vi "Error Query.vi"(8 "error in (no error)":errorcluster, 11 "VISA resource name":refnum<visa-resource-name>) -> (0 "error out":errorcluster, 1 "Error Message":string, 2 "Error Code":i32[](array[numeric]), 3 "VISA resource name out":refnum<visa-resource-name>)   [LabVIEW 2025]
doc: "Queries the instrument for any errors in the instrument's error queue. It will continue to read errors until all errors have been read from the instrument. Any errors will be returned in the <B>error out</B> control.\n\n<B>Note:</B>\nThis VI is called automatically by most driver VIs so it is not usually necessary to call this in an application."
panel:
  # "EDIT: Note: The Error Query VI is included as a subVI in all driver VIs except low-level API VIs. If the instrument does not support error query, then remove the VI and remove subVI calls in each instrument driver VI that calls it."
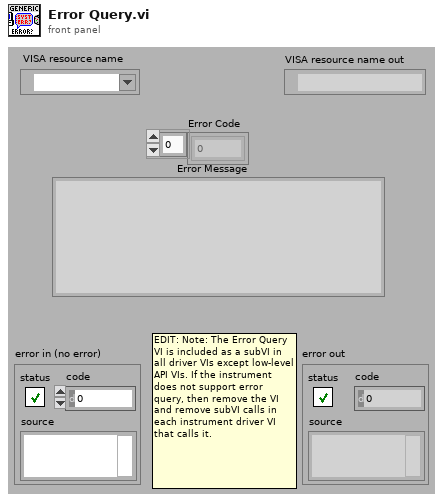
[diagram p1: front panel]
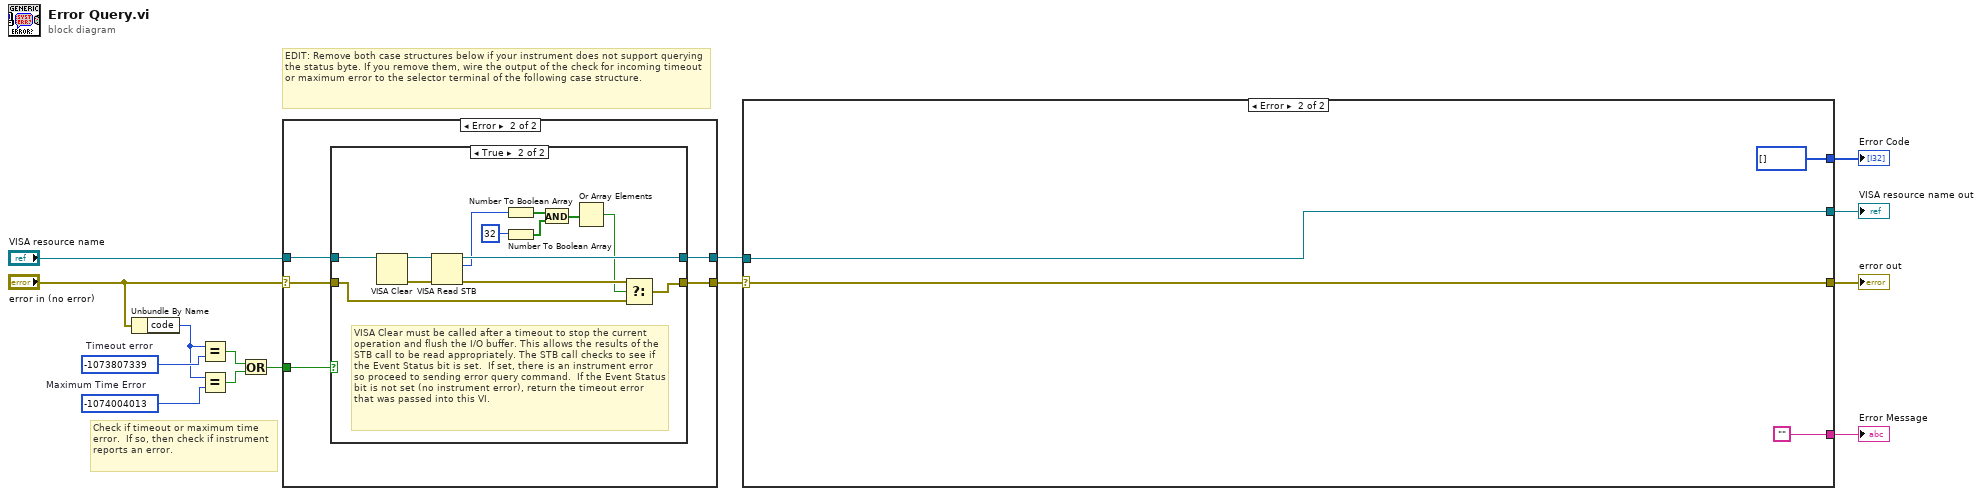
[diagram p0: block diagram]
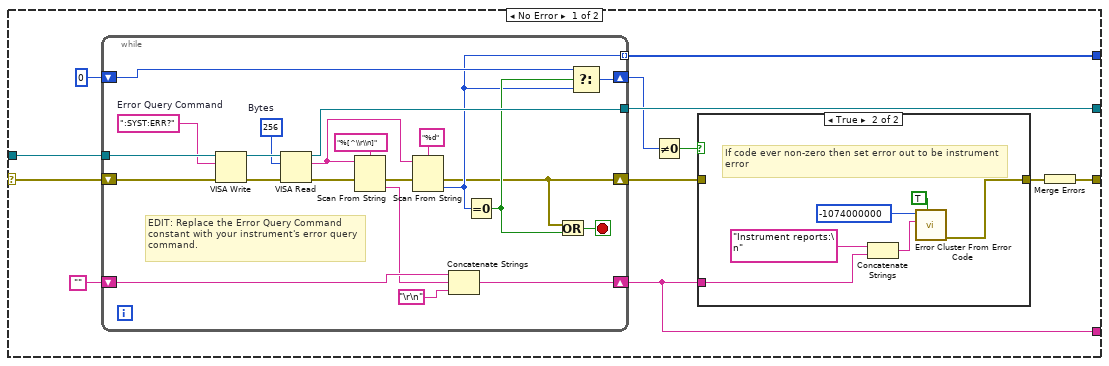
[diagram p4: hidden frame]
diagram:
  w5 = -1074004013  # Maximum Time Error
  w7 = -1073807339  # Timeout error
  # "Check if timeout or maximum time error.  If so, then check if instrument reports an error."
  # "EDIT: Remove both case structures below if your instrument does not support querying the status byte. If you remove them, wire the output of the check for incoming timeout or maximum error to the selector terminal of the following case structure."
  n1 = Unbundle By Name("error in (no error)") -> ("code"=w6:i32)
  n2 = Equal?(x=w6, y=w7) -> (x = y?=w3:bool)
  n3 = Equal?(x=w6, y=w5) -> (x = y?=w4:bool)
  n4 = Or(x=w3, y=w4) -> (x .or. y?=w2:bool)
  n5 = case shown="Error" "error in (no error)" {
    selector: "error in (no error)" -> [w15 w19]
    tunnel: "VISA resource name" -> [w16 w21]
    tunnel: [w16 w20] -> w9
    tunnel: [w15 w18] -> w10
    tunnel: w2 -> [_ w17]
    frame No Error {
    }
    frame Error {
      n6 = case shown="True" w17 {
        tunnel: w21 -> [w23 w30]
        tunnel: [w23 w27] -> w20
        tunnel: w19 -> [w22 w32]
        tunnel: [w22 w31] -> w18
        frame False {
          # "Error code not a timeout, so best to pass on to user."
        }
        frame True {
          # "VISA Clear must be called after a timeout to stop the current operation and flush the I/O buffer. This allows the results of the  STB call to be read appropriately. The STB call checks to see if the Event Status bit is set.  If set, there is an instrument error so proceed to sending error query command.  If the Event Status bit is not set (no instrument error), return the timeout error that was passed into this VI."
          n7 = VISA Clear(VISA resource name=w30) -> (VISA resource name out=w29:refnum<visa-resource-name>, error out=w28:errorcluster)  [unwired: 1 in]
          n8 = VISA Read STB(8:w28, 11:w29) -> (0:w26:errorcluster, 2:w25:u16, 3:w27:refnum<visa-resource-name>)
          n9 = Number To Boolean Array(number=w25) -> (Boolean array=w33:bool[])
          n10 = Number To Boolean Array(number=32) -> (Boolean array=w35:bool[])
          n11 = And(x=w33, y=w35) -> (x .and. y?=w34:bool[])
          n12 = Or Array Elements(Boolean array=w34) -> (logical OR=w24:bool)
          n13 = Select(t=w26, s=w24, f=w32) -> (s? t:f=w31:errorcluster)
        }
      }
    }
  }
  n14 = case shown="Error" w10 {
    selector: w10 -> [w38 w78]
    tunnel: [w48 w81] -> w14
    tunnel: w9 -> [w47 w81]
    tunnel: [w45 w78] -> w13
    tunnel: [w37 ""] -> w12
    tunnel: [w40 i32[] []] -> w11
    frame No Error {
      n15 = while {
        tunnel: [w77] -> w48
        tunnel: w47 -> [w76]
        shift-right: [w64] -> w37
        shift-left: "" -> [w67]
        shift-right: [w62] -> w41
        shift-left: 0 -> [w63]
        shift-right: [w56] -> w39
        shift-left: w38 -> [w61]
        tunnel: [w57] -> w40 mode=indexing
        stop <- w70 stop-if-true
        w74 = u32 256  # Bytes
        w72 = ":SYST:ERR?"  # Error Query Command
        # "EDIT: Replace the Error Query Command constant with your instrument's error query command."
        n16 = VISA Write(VISA resource name=w76, write buffer=w72, error in (no error)=w61) -> (VISA resource name out=w75:refnum<visa-resource-name>, error out=w73:errorcluster)  [unwired: 1 out]
        n17 = VISA Read(VISA resource name=w75, byte count=w74, error in (no error)=w73) -> (VISA resource name out=w77:refnum<visa-resource-name>, read buffer=w68:string, error out=w60:errorcluster)  [unwired: 1 out]
        n18 = Scan From String(format string="%[^\\r\\n]", input string=w68, error in=w60) -> (error out=w59:errorcluster, output 1=w65:string)  [unwired: 2 in, 2 out]
        n19 = Scan From String(format string="%d", input string=w68, error in=w59) -> (error out=w56:errorcluster, output 1=w57:i32)  [unwired: 2 in, 2 out]
        n20 = Concatenate Strings(w67, w65, "\r\n") -> (w64:string)
        n21 = Equal To 0?(x=w57) -> (x = 0?=w58:bool)
        n22 = Or(x=w56, y=w58) -> (x .or. y?=w70:bool)
        n23 = Select(t=w63, s=w58, f=w57) -> (s? t:f=w62:i32)
      }
      n24 = Not Equal To 0?(x=w41) -> (x != 0?=w43:bool)
      n25 = case shown="True" w43 {
        tunnel: w37 -> [_ w54]
        tunnel: [w49 w50] -> w42
        tunnel: w39 -> [w49 _]
        frame False {
        }
        frame True {
          # "If code ever non-zero then set error out to be instrument error"
          n26 = Concatenate Strings("Instrument reports:\n" ("Source"), w54) -> (w51:string)
          n27 = call <vilib>:"Error Cluster From Error Code.vi"("show call chain? (False)"=TRUE, "error message (\"\")"=w51, "error code (0)"=-1074000000 ("Code")) -> ("error out"=w50:errorcluster)  [unwired: 6 in]
        }
      }
      n28 = Merge Errors(w42) -> (w45:errorcluster)
    }
    frame Error {
    }
  }
  "VISA resource name out" <- w14
  "error out" <- w13
  "Error Message" <- w12
  "Error Code" <- w11
